vi "GetQueueValue.vi"(3 "error in":errorcluster, 4 "vi name":string, 5 "Q":refnum<queue>[](array[refnum])) -> (0 "error out":errorcluster, 2 "Queue out":refnum<queue>)   [LabVIEW 2018]
doc: "Checks for errors in the queue"
uses:
  <userlib>/ROS for LabVIEW Software/ROS/Code/_ROSDefinition.vi
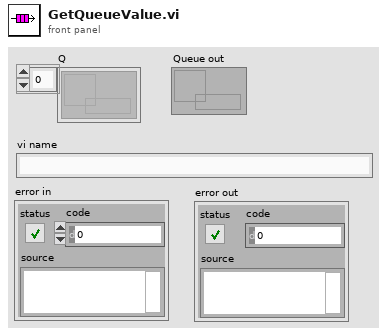
[diagram p1: front panel]
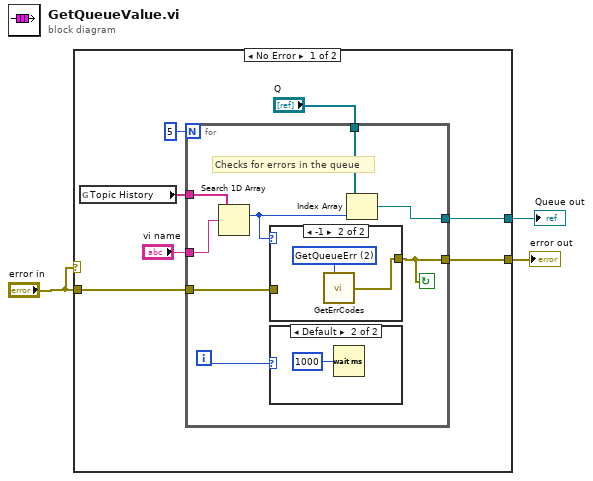
[diagram p0: block diagram]
diagram:
  n1 = case shown="No Error" "error in" {
    tunnel: [w8 w23] -> w3
    tunnel: [w7 _] -> w2
    tunnel: "error in" -> [w4 w23]
    frame No Error {
      n2 = global read "_ROSDefinition.vi" "Topic History"() -> (w5:string[])
      n3 = for {
        N: 5 -> [_]
        tunnel: "vi name" -> [w11]
        tunnel: [w17] -> w7
        tunnel: [w16] -> w8
        tunnel: "Q" -> [w14]
        tunnel: w5 -> [w13]
        tunnel: w4 -> [w12]
        i -> [w15]
        stop <- w16 continue-if-true
        # "Checks for errors in the queue"
        n4 = Search 1D Array(1D array=w13, element=w11) -> (index of element=w18:i32)  [unwired: 1 in]
        n5 = case shown="-1" w18 {
          tunnel: [w20 w21] -> w16
          tunnel: w12 -> [w20 _]
          frame Default {
          }
          frame -1 {
            w22 = u16 2 items=["TopicReadTimeout", "Read=SS", "GetQueueErr"] ("Error")
            n6 = call <userlib>:"GetErrCodes.vi"("Error"=w22) -> ("Error"=w21:errorcluster)  [unwired: 1 in]
          }
        }
        n7 = case shown="Default" w15 {
          frame 0 {
          }
          frame Default {
            n8 = Wait (ms)(milliseconds to wait=u32 1000) -> ()  [unwired: 1 out]
          }
        }
        n9 = Index Array(array=w14, index=w18) -> (element=w17:refnum<queue>)
      }
    }
    frame Error {
    }
  }
  "error out" <- w3
  "Queue out" <- w2
